vi "NyquistTrimCoefficients.vi"(6 "Coherence":dbl[](array[numeric]), 7 "Cutoff type":string(combo), 8 "InterpolatedPhase":dbl[](array[numeric]), 9 "InterpolatedCoefficients":dbl[](array[numeric]), 10 "Frequencies":dbl[](array[numeric]), 11 "fcut (Hz)":dbl) -> (0 "NyquistLimitedPhase":dbl[](array[numeric]), 1 "NyquistLimitedCoefficients":dbl[](array[numeric]), 2 "NyquistLimitedFrequency":dbl[](array[numeric]), 3 "fcut Index":dbl, 4 "NyquistLimitedCoherence":dbl[](array[numeric]))   [LabVIEW 2016]
uses:
  <vilib>/Analysis/NI_AALBase.lvlib
panel:
  in  "cosineFadeLength":i32=12
  out "XY Graph":cluster{"Frequencies":dbl[], dbl[]}[](graph)
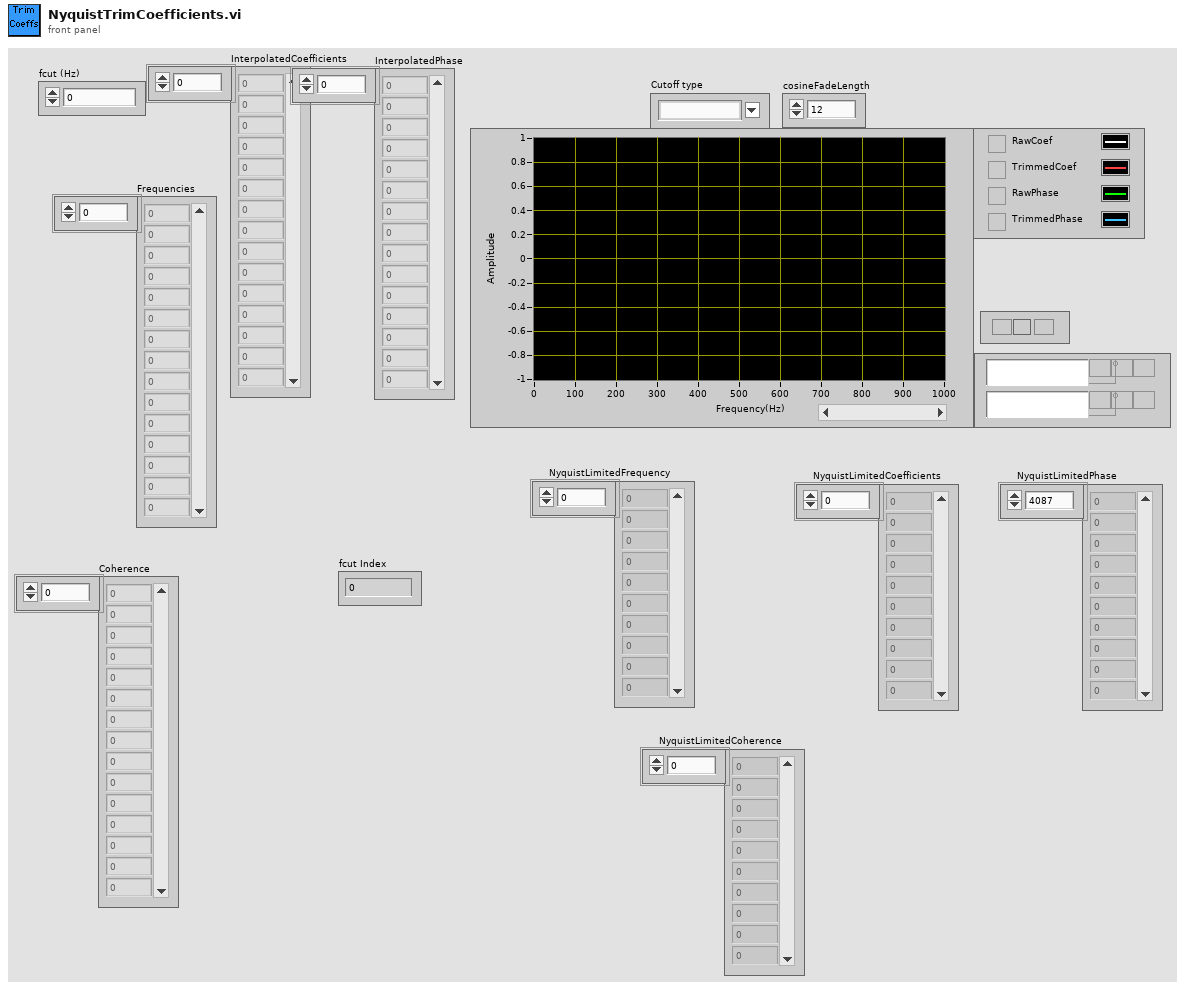
[diagram p1: front panel]
types:
  T1 = cluster{"Frequencies":dbl[], "InterpolatedCoefficients":dbl[]}
  T2 = cluster{"Frequencies":dbl[], "InterpolatedPhase":dbl[]}
  T3 = cluster{"Frequencies":dbl[], "InterpolatedPhase":dbl[]}[]
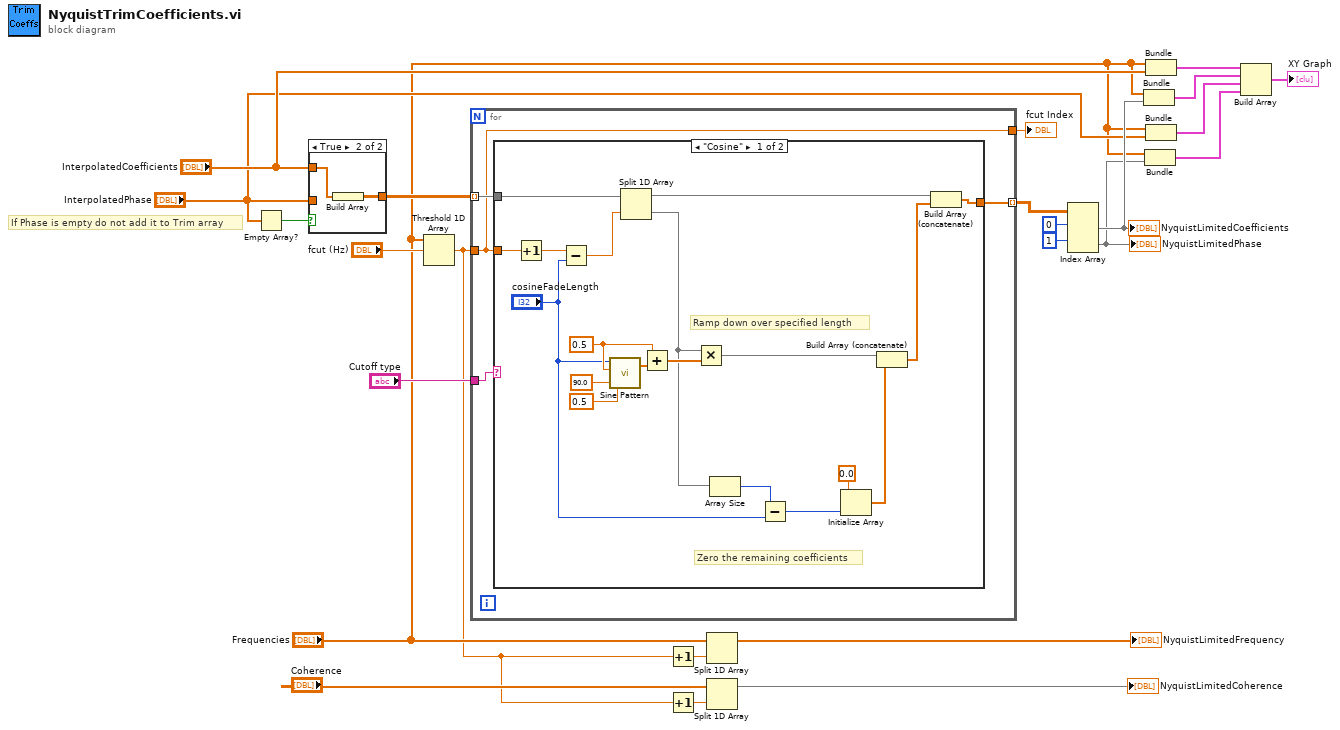
[diagram p0: block diagram]
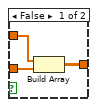
[diagram p2: hidden frame]
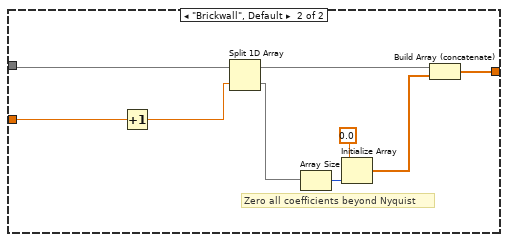
[diagram p3: hidden frame]
diagram:
  # "If Phase is empty do not add it to Trim array"
  n1 = Empty Array?(array="InterpolatedPhase") -> (empty?=w10:bool)
  n2 = case shown="True" w10 {
    tunnel: "InterpolatedCoefficients" -> [w27 w29]
    tunnel: [w26 w28] -> w12
    tunnel: "InterpolatedPhase" -> [w25 _]
    frame False {
      n3 = Build Array(w27, w25) -> (w26:dbl[][])
    }
    frame True {
      n4 = Build Array(w29) -> (w28:dbl[][])
    }
  }
  n5 = Threshold 1D Array(2:"fcut (Hz)", 3:"Frequencies") -> (0:w2:dbl)  [unwired: 1 in]
  n6 = for {
    tunnel: "Cutoff type" -> [w33]
    tunnel: w2 -> [w30]
    tunnel: [w32] -> w8 mode=indexing
    tunnel: w12 -> [w31] mode=indexing
    tunnel: [w30] -> w9
    n7 = case shown="\"Cosine\"" w33 {
      tunnel: w31 -> [w42 w59]
      tunnel: [w41 w55] -> w32
      tunnel: w30 -> [w35 w54]
      frame "Cosine" {
        w49 = 0.5 ("amplitude")
        # "Ramp down over specified length"
        # "Zero the remaining coefficients"
        n8 = Increment(x=w35) -> (x+1=w34:dbl)
        n9 = Subtract(x=w34, y="cosineFadeLength") -> (x-y=w40:dbl)
        n10 = call <vilib>:"Sine Pattern.vi"("cycles"=0.5, "phase(degrees)"=90.0, "amplitude"=w49, "samples"="cosineFadeLength") -> ("Sinusoidal Pattern"=w51:dbl[])  [unwired: 1 out]
        n11 = Split 1D Array(array=w42, index=w40) -> (first subarray=w43:dbl[], second subarray=w36:dbl[])
        n12 = Add(x=w49, y=w51) -> (x+y=w39:dbl[])
        n13 = Multiply(x=w36, y=w39) -> (x*y=w47:dbl[])
        n14 = Array Size(array=w36) -> (size(s)=w46:i32)
        n15 = Subtract(x=w46, y="cosineFadeLength") -> (x-y=w45:i32)
        n16 = Initialize Array(0.0 ("element"), w45) -> (w44:dbl[])
        n17 = Build Array (concatenate)(w47, w44) -> (w38:dbl[])
        n18 = Build Array (concatenate)(w43, w38) -> (w41:dbl[])
      }
      frame "Brickwall", Default {
        # "Zero all coefficients beyond Nyquist"
        n19 = Increment(x=w54) -> (x+1=w53:dbl)
        n20 = Split 1D Array(array=w59, index=w53) -> (first subarray=w56:dbl[], second subarray=w58:dbl[])
        n21 = Array Size(array=w58) -> (size(s)=w61:i32)
        n22 = Initialize Array(0.0 ("element"), w61) -> (w57:dbl[])
        n23 = Build Array (concatenate)(w56, w57) -> (w55:dbl[])
      }
    }
  }
  "fcut Index" <- w9
  n24 = Increment(x=w2) -> (x+1=w6:dbl)
  n25 = Increment(x=w2) -> (x+1=w4:dbl)
  n26 = Split 1D Array(array="Frequencies", index=w6) -> (first subarray=→"NyquistLimitedFrequency":dbl[])  [unwired: 1 out]
  n27 = Split 1D Array(array="Coherence", index=w4) -> (first subarray=→"NyquistLimitedCoherence":dbl[])  [unwired: 1 out]
  n28 = Index Array(array=w8, index (row) #1=0 ("index (row)"), index (row) #2=1 ("index (row)")) -> (element #1=w18:dbl[], element #2=w16:dbl[])  [unwired: 2 in]
  "NyquistLimitedCoefficients" <- w18
  "NyquistLimitedPhase" <- w16
  n29 = Bundle("Frequencies"="Frequencies", w18) -> (w17:cluster{"Frequencies":dbl[], dbl[]})  [unwired: 1 in]
  n30 = Bundle("Frequencies"="Frequencies", w16) -> (w14:cluster{"Frequencies":dbl[], dbl[]})  [unwired: 1 in]
  n31 = Bundle("Frequencies"="Frequencies", "InterpolatedCoefficients"="InterpolatedCoefficients") -> (w19:T1)  [unwired: 1 in]
  n32 = Bundle("Frequencies"="Frequencies", "InterpolatedPhase"="InterpolatedPhase") -> (w15:T2)  [unwired: 1 in]
  n33 = Build Array(w19, w17, w15, w14) -> (→"XY Graph":T3)
